vi "LoadTiming Parameters.vi"(3 "error in (no error)":errorcluster, 4 "refnum":T2, 5 "Input Cluster":T1, 6 "section":string) -> (0 "error out":errorcluster, 1 "refnum out":T2, 2 "Output Cluster":T1)   [LabVIEW 2009]
uses:
  <vilib>/Utility/config.llb/Config Data RefNum.ctl
  Timing Parameters.ctl
  <vilib>/Utility/config.llb/Read Key (Double).vi
  <vilib>/Utility/config.llb/NI_LVConfig.lvlib
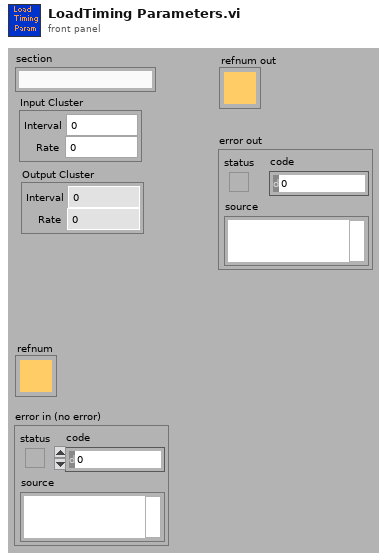
[diagram p1: front panel]
types:
  T1 = typedef "Timing Parameters.ctl" = cluster{"Interval":dbl, "Rate ":dbl}
  T2 = typedef "NI_LVConfig.lvlib/Config Data RefNum.ctl" = refnum<k1>
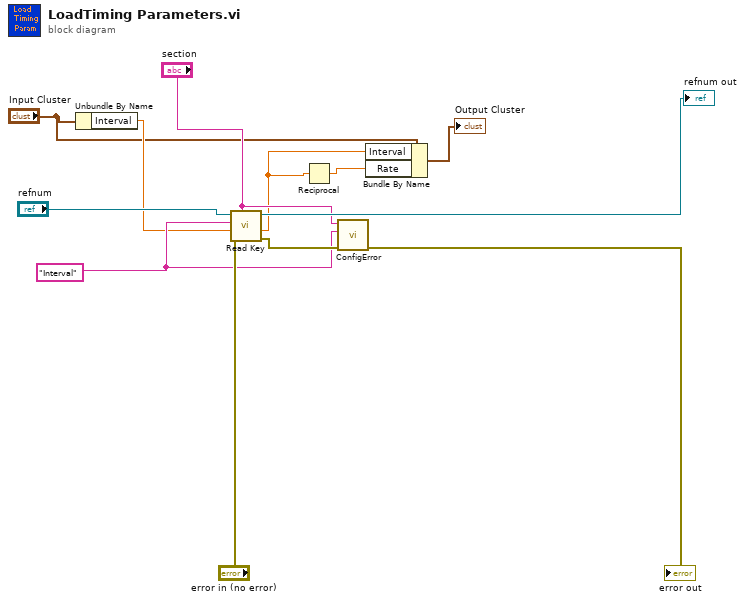
[diagram p0: block diagram]
diagram:
  w7 = "Interval" ("key")
  n1 = Unbundle By Name("Input Cluster") -> ("Interval"=w5:dbl)
  n2 = call-poly <vilib>:"Read Key.vi"("section"="section", "error in (no error)"="error in (no error)", "default value"=w5, "key"=w7, "refnum"="refnum") -> ("error out"=w9:errorcluster, "value"=w2:dbl, "refnum out"=→"refnum out":T2)  [unwired: 4 out]
  n3 = Reciprocal(x=w2) -> (1/x=w1:dbl)
  n4 = call "ConfigError.vi"("error in (no error)"=w9, "Key"=w7, "Section"="section") -> ("error out"=→"error out":errorcluster)  [unwired: 8 out]
  n5 = Bundle By Name(cluster="Input Cluster", "Interval"=w2, "Rate"=w1) -> (→"Output Cluster":T1)
